vi "LJLogUD(old).vi"() -> ()   [LabVIEW 2020]
panel:
  in  "Change Working Directory":bool
  in  "Max File Size (Bytes)":i32=1048576 min=1 max=2000000000
  in  "Graph?":bool[](array[boolean])
  out "Waveform Graph":cluster{dbl, dbl, dbl[][]}(graph)
  in  "Graph History":i32=1000 min=0
  out "Address":string
  out "Device Type":string
  in  "Ranges":u16[](array[ring])=[0, 0, 0, 0, 0, 0, 0, 0] items=["LJ_rgBIP10V", "LJ_rgBIP5V", "LJ_rgUNI5V", "LJ_rgUNI2P5V", "LJ_rgUNI1P25V", "LJ_rgBIP1V", "LJ_rgUNIP625V", "LJ_rgBIPP1V", "LJ_rgBIPP01V"]
  in  "SettlingFactor":u8
  in  "Resolution":u8
  in  "exit":bool
  out "Scaled":dbl[](array[numeric]) format="%.6f"
  in  "Scaling Equation":string[](array[string])=["y=v0", "y=v1", "y=v2", "y=v3", "y=v4", "y=v5", "y=v6", "y=v7"]
  in  "# Channels":i32=4 min=1
  in  "-Ch":string[](array[string])=["31", "31", "31", "31", "31", "31", "31", "31"]
  out "Voltage":dbl[](array[numeric]) format="%.6f"
  in  "+Ch":string[](array[string])=["0", "1", "2", "3", "4", "5", "6", "7"]
  out "# of iterations":i32
  in  "Interval (ms)":u32=500
  out "Current Data File":path
  in  "Data File Prefix":string="data"
  in  "Write To File":bool
  out "Error Message":string
  # "0"
  # "1"
  # "2"
  # "3"
  # "4"
  # "5"
  # "6"
  # "7"
  # "8"
  # "9"
  # "10"
  # "11"
  # "12"
  # "13"
  # "14"
  # "15"
  # "-\"a\" - \"p\" correspond to the raw Voltage value\n  from the 1st through 16th row.\n-The scaled output value is \"y\".\n-If your equation has an error, the output\n  will be zero."
  # "# scans"
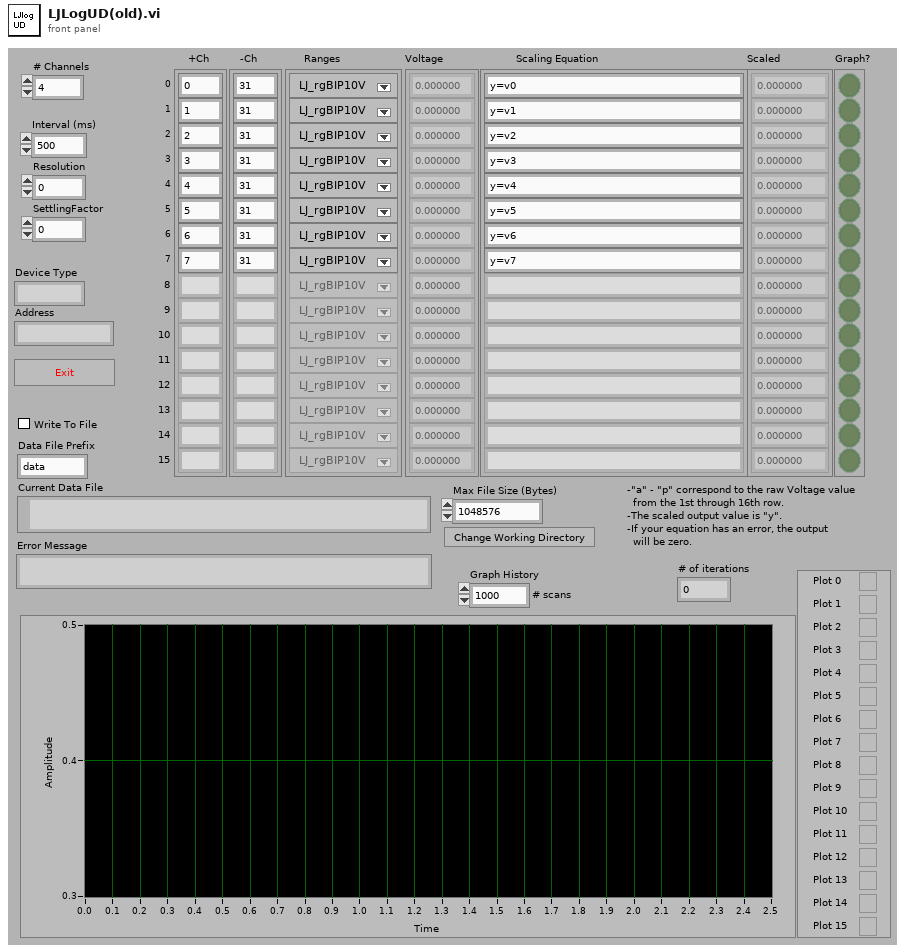
[diagram p1: front panel]
types:
  T1 = cluster{"+Ch":string[], "-Ch":string[], "Ranges":u16[], "Scaling Equation":string[], "Graph?":bool[]}
  T2 = cluster{"# Channels":i32, "+Ch":string[], "-Ch":string[], "Ranges":u16[], "Scaling Equation":string[]}
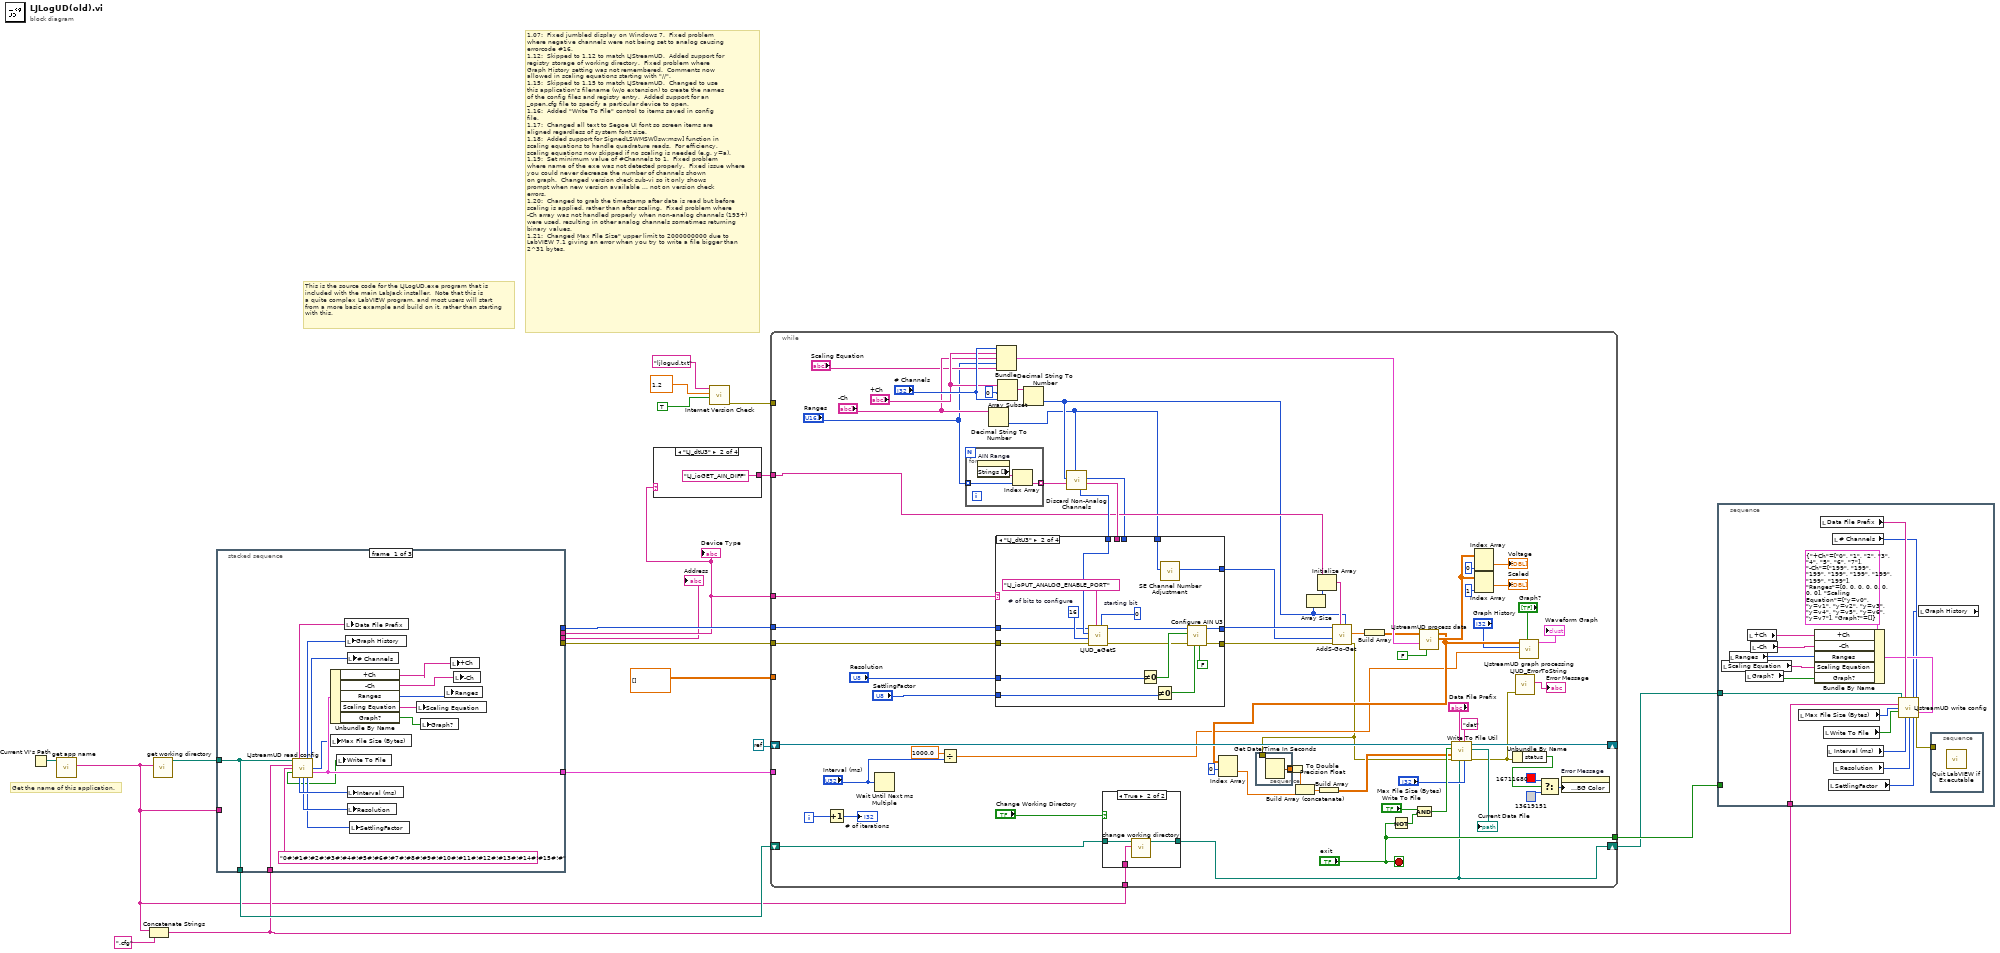
[diagram p0: block diagram]
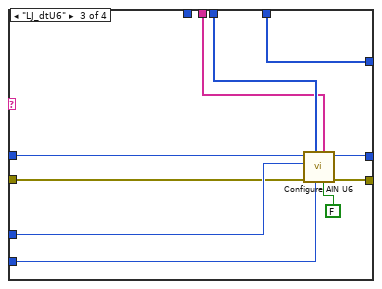
[diagram p4: hidden frame]
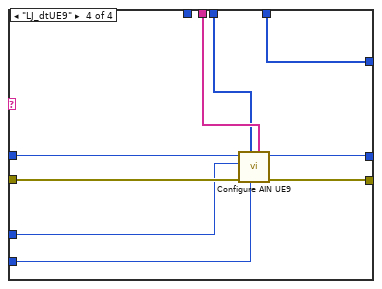
[diagram p5: hidden frame]
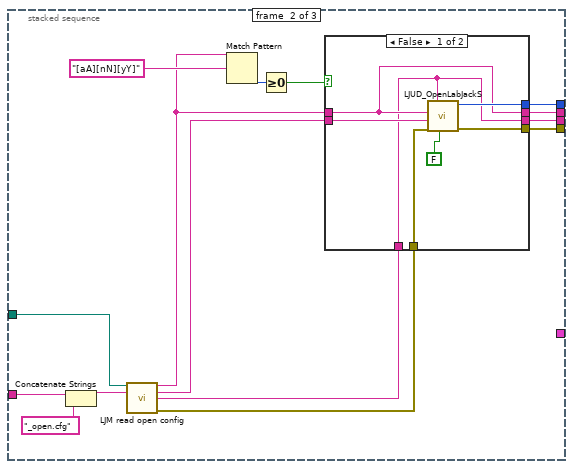
[diagram p6: hidden frame]
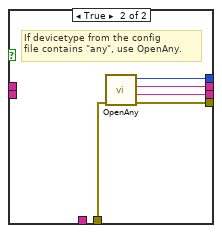
[diagram p7: hidden frame]
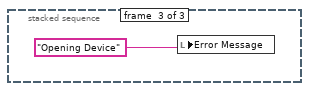
[diagram p8: hidden frame]
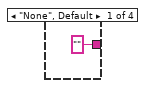
[diagram p9: hidden frame]
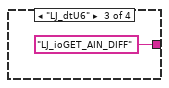
[diagram p10: hidden frame]
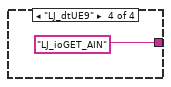
[diagram p11: hidden frame]
diagram:
  # "This is the source code for the LJLogUD.exe program that is\nincluded with the main LabJack installer.  Note that this is \na quite complex LabVIEW program, and most users will start\nfrom a more basic example and build on it, rather than starting\nwith this."
  # "Get the name of this application."
  # "1.07:  Fixed jumbled display on Windows 7.  Fixed problem\nwhere negative channels were not being set to analog causing\nerrorcode #16.\n1.12:  Skipped to 1.12 to match LJStreamUD.  Added support for\nregistry storage of working directory.  Fixed problem where\nGraph History setting was not remembered.  Comments now\nallowed in scaling equations starting with \"//\".\n1.15:  Skipped to 1.15 to match LJStreamUD.  Changed to use\nthis application's filename (w/o extension) to create the names\nof the config files and registry entry.  Added support for an\n_open.cfg file to specify a particular device to open.\n1.16:  Added \"Write To File\" control to items saved in config\nfile.\n1.17:  Changed all text to Segoe UI font so screen items are\naligned regardless of system font size.\n1.18:  Added support for SignedLSWMSW[lsw:msw] function in\nscaling equations to handle quadrature reads.  For efficiency,\nscaling equations now skipped if no scaling is needed (e.g. y=a).\n1.19:  Set minimum value of #Channels to 1.  Fixed problem\nwhere name of the exe was not detected properly.  Fixed issue where\nyou could never decrease the number of channels shown\non graph.  Changed version check sub-vi so it only shows\nprompt when new version available ... not on version check\nerrors.\n1.20:  Changed to grab the timestamp after data is read but before\nscaling is applied, rather than after scaling.  Fixed problem where\n-Ch array was not handled properly when non-analog channels (193+)\nwere used, resulting in other analog channels sometimes returning\nbinary values.\n1.21:  Changed Max File Size\" upper limit to 2000000000 due to\nLabVIEW 7.1 giving an error when you try to write a file bigger than\n2^31 bytes."
  n1 = Current VI's Path() -> (path=w1:path)
  n2 = call "get app name.vi"("Current VI's Path"=w1) -> ("App Name Without Extension"=w2:string)  [unwired: 4 in, 2 out]
  n3 = Concatenate Strings(w2, ".cfg" ("filename")) -> (w7:string)
  n4 = call "get working directory.vi"("Application Name"=w2) -> ("Working Directory"=w11:path)  [unwired: 9 in, 1 out]
  n5 = stacked-sequence {
    tunnel: [w37 _ _] -> w17
    tunnel: [w24 _ _] -> w10
    tunnel: w11 -> [w24 w38 _]
    tunnel: w7 -> [w23 _ _]
    tunnel: w2 -> [_ w51 _]
    tunnel: [_ w49 _] -> w6
    tunnel: [_ w48 _] -> w5
    tunnel: [_ w47 _] -> w4
    tunnel: [_ w46 _] -> w3
    frame #0 {
      n6 = call "LJstreamUD read config.vi"("Working Directory"=w24, "filename"=w23, "ChP Default"="0#!#1#!#2#!#3#!#4#!#5#!#6#!#7#!#8#!#9#!#10#!#11#!#12#!#13#!#14#!#15#!#") -> ("Data File Prefix"=w32:string, "Graph History"=w26:i32, "# Channels"=w28:i32, "Max File Size (Bytes)"=w25:i32, "Write To File"=w21:bool, "Channel Setup"=w37:T1, "Interval (ms)"=w31:u32, "Resolution"=w30:u8, "SettlingFactor"=w29:u8)  [unwired: 4 out]
      n7 = Unbundle By Name(w37) -> ("+Ch"=w33:string[], "-Ch"=w34:string[], "Ranges"=w35:u16[], "Scaling Equation"=w36:string[], "Graph?"=w27:bool[])
      n8 = local write "Max File Size (Bytes)"(w25) -> ()
      n9 = local write "Write To File"(w21) -> ()
      n10 = local write "Data File Prefix"(w32) -> ()
      n11 = local write "Graph History"(w26) -> ()
      n12 = local write "# Channels"(w28) -> ()
      n13 = local write "Interval (ms)"(w31) -> ()
      n14 = local write "Resolution"(w30) -> ()
      n15 = local write "SettlingFactor"(w29) -> ()
      n16 = local write "Scaling Equation"(w36) -> ()
      n17 = local write "Graph?"(w27) -> ()
      n18 = local write "Ranges"(w35) -> ()
      n19 = local write "+Ch"(w33) -> ()
      n20 = local write "-Ch"(w34) -> ()
    }
    frame #1 {
      n21 = Concatenate Strings(w51, "_open.cfg" ("filename")) -> (w50:string)
      n22 = call "LJM read open config.vi"("Working Directory"=w38, "filename"=w50) -> ("DeviceType"=w41:string, "ConnectionType"=w40:string, "Identifier"=w42:string, "error out"=w39:errorcluster)  [unwired: 10 in]
      n23 = Match Pattern(string=w41, regular expression="[aA][nN][yY]") -> (offset past match=w45:i32)  [unwired: 1 in, 3 out]
      n24 = Greater Or Equal To 0?(x=w45) -> (x >= 0?=w43:bool)
      n25 = case shown="False" w43 {
        tunnel: [w59 w64] -> w49
        tunnel: [w55 w63] -> w48
        tunnel: [w53 w62] -> w47
        tunnel: [w58 w61] -> w46
        tunnel: w42 -> [w53 _]
        tunnel: w41 -> [w55 _]
        tunnel: w40 -> [w54 _]
        tunnel: w39 -> [w56 w60]
        frame False {
          n26 = call "LJUD_OpenLabJackS.vi"("FirstFound"=FALSE, "Address"=w53, "error in"=w56, "ConnectionType"=w54, "DeviceType"=w55) -> ("error out"=w58:errorcluster, "Handle"=w59:i32)  [unwired: 4 in, 1 out]
        }
        frame True {
          # "If devicetype from the config\nfile contains \"any\", use OpenAny."
          n27 = call "OpenAny.vi"("error in"=w60) -> ("error out"=w61:errorcluster, "Address Found"=w62:string, "Device Type Found"=w63:string, "Handle"=w64:i32)  [unwired: 7 in]
        }
      }
    }
    frame #2 {
      n28 = local write "Error Message"("Opening Device" ("Error Message")) -> ()
    }
  }
  "Device Type" <- w5
  "Address" <- w4
  n29 = case shown="\"LJ_dtU3\"" w5 {
    tunnel: ["" ("IOType") "LJ_ioGET_AIN_DIFF" ("IOType") "LJ_ioGET_AIN_DIFF" ("IOType") "LJ_ioGET_AIN" ("IOType")] -> w19
    frame "None", Default {
    }
    frame "LJ_dtU3" {
    }
    frame "LJ_dtU6" {
    }
    frame "LJ_dtUE9" {
    }
  }
  n30 = call "Internet Version Check.vi"("Prompt If Newer Version Available"=TRUE, "Version In"=1.2, "Version File Name"="ljlogud.txt") -> ("error out"=w13:errorcluster)  [unwired: 6 in, 2 out]
  n31 = while {
    shift-left: w10 -> [w73]
    shift-right: [w72] -> w9
    tunnel: w2 -> [w74]
    tunnel: w13 -> [_]
    tunnel: dbl[][] [] ("Waveform Chart") -> [_]
    tunnel: w19 -> [w100]
    tunnel: w3 -> [w101]
    tunnel: w5 -> [w113]
    tunnel: w6 -> [w112]
    shift-left: refnum<k0> refnum -> [w122]
    shift-right: [w124] -> _
    tunnel: w17 -> [_]
    tunnel: ["exit"] -> w12
    i -> [w129]
    stop <- "exit" stop-if-true
    n32 = Increment(x=w129) -> (x+1=→"# of iterations":i32)
    n33 = Wait Until Next ms Multiple(millisecond multiple="Interval (ms)") -> ()  [unwired: 1 out]
    n34 = Divide(x=1000.0, y="Interval (ms)") -> (x/y=w85:dbl)
    n35 = for {
      tunnel: "Ranges" -> [w184] mode=indexing
      tunnel: [w183] -> w130 mode=indexing
      n36 = property on="AIN Range" class="Ring (strict)"() -> ("Strings []"=w185:string[])  [unwired: 2 in, 2 out]
      n37 = Index Array(array=w185, index=w184) -> (element=w183:string)
    }
    n38 = Decimal String To Number(string="-Ch") -> (number=w70:i32[])  [unwired: 2 in, 1 out]
    n39 = Bundle("# Channels"="# Channels", "+Ch"="+Ch", "-Ch"="-Ch", "Ranges"="Ranges", "Scaling Equation"="Scaling Equation") -> (w117:T2)  [unwired: 1 in]
    n40 = Array Subset(array="+Ch", index=0 ("Array Index"), length="# Channels") -> (w131:string[])
    n41 = Decimal String To Number(string=w131) -> (number=w81:i32[])  [unwired: 2 in, 1 out]
    n42 = call "Discard Non-Analog Channels.vi"("Channels In (-)"=w70, "Ranges In"=w130, "Channels In"=w81) -> ("Ranges Out"=w110:string[], "Channels Out"=w82:i32[], "FIO/EIO Analog Enable"=w111:i32)  [unwired: 5 in, 1 out]
    n43 = case shown="\"LJ_dtU3\"" w113 {
      tunnel: w111 -> [_ w152 _ _]
      tunnel: w101 -> [w146 w151 w165 w181]
      tunnel: w112 -> [w145 w150 w166 w182]
      tunnel: [w146 w158 w172 w177] -> w106
      tunnel: [w145 w159 w173 w178] -> w104
      tunnel: w110 -> [_ _ w170 w180]
      tunnel: w82 -> [_ _ w171 w179]
      tunnel: "Resolution" -> [_ w163 w169 w176]
      tunnel: "SettlingFactor" -> [_ w161 w168 w175]
      tunnel: [w144 w157 w164 w174] -> w103
      tunnel: w70 -> [w144 w147 w164 w174]
      frame "None", Default {
      }
      frame "LJ_dtU3" {
        w154 = 0  # starting bit
        w155 = 16  # # of bits to configure
        n44 = call "LJUD_eGetS.vi"("Channel"=w154, "IOType"="LJ_ioPUT_ANALOG_ENABLE_PORT" ("Channel"), "error in"=w151, "x1"=w155, "Value Write"=w152, "Handle In"=w150) -> ("error out"=w149:errorcluster, "Handle Out"=w148:i32)  [unwired: 3 in, 1 out]
        n45 = Not Equal To 0?(x=w163) -> (x != 0?=w162:bool)
        n46 = Not Equal To 0?(x=w161) -> (x != 0?=w160:bool)
        n47 = call "SE Channel Number Adjustment.vi"("Channels In"=w147) -> ("Channels Out"=w157:i32[])  [unwired: 10 in]
        n48 = call "Configure AIN U3.vi"("Binary"=FALSE ("Enable DAC1"), "longSettling"=w160, "error in"=w149, "quickSample"=w162, "Handle In"=w148) -> ("error out"=w158:errorcluster, "Handle Out"=w159:i32)  [unwired: 5 in]
      }
      frame "LJ_dtU6" {
        n49 = call "Configure AIN U6.vi"("Binary"=FALSE ("Enable Counter0"), "Ranges"=w170, "SettlingFactor"=w168, "Positive Channels"=w171, "error in"=w165, "Resolution"=w169, "Handle In"=w166) -> ("error out"=w172:errorcluster, "Handle Out"=w173:i32)  [unwired: 3 in]
      }
      frame "LJ_dtUE9" {
        n50 = call "Configure AIN UE9.vi"("Ranges"=w180, "SettlingFactor"=w175, "Channels"=w179, "error in"=w181, "Resolution"=w176, "Handle In"=w182) -> ("error out"=w177:errorcluster, "Handle Out"=w178:i32)  [unwired: 4 in]
      }
    }
    n51 = case shown="True" "Change Working Directory" {
      tunnel: w74 -> [_ w141]
      tunnel: w73 -> [w138 w140]
      tunnel: [w138 w139] -> w72
      frame False {
      }
      frame True {
        n52 = call "change working directory.vi"("Application Name"=w141, "Working Directory In"=w140) -> ("Working Directory Out"=w139:path)  [unwired: 9 in]
      }
    }
    n53 = Array Size(array=w81) -> (size(s)=w115:i32)
    n54 = Initialize Array(w100, w115) -> (w114:string[])
    n55 = call "AddS-Go-Get.vi"("Channels"=w81, "IOTypes"=w114, "error in"=w106, "x1"=w103, "Handle In"=w104) -> ("error out"=w71:errorcluster, "Values Read"=w105:dbl[])  [unwired: 4 in, 1 out]
    n56 = stacked-sequence {
      tunnel: [w143] -> w99
      tunnel: w71 -> [_]
      frame #0 {
        n57 = Get Date/Time In Seconds() -> (seconds since 1Jan1904=w142:timestamp)
        n58 = To Double Precision Float(number=w142) -> (double precision float=w143:dbl)
      }
    }
    n59 = Build Array(w105) -> (w97:dbl[][])
    n60 = Not(x="exit") -> (.not. x?=w133:bool)
    n61 = And(x="Write To File", y=w133) -> (x .and. y?=w123:bool)
    n62 = call "LJstreamUD process data.vi"("Disable Scaling"=FALSE, "Channel Config"=w117, "Voltages"=w97) -> ("Volts,Scaled Averages"=w116:dbl[][], "Scaled Data"=w90:dbl[][])  [unwired: 7 in]
    n63 = Index Array(array=w90, index (row)=0 ("Index (row)")) -> (element=w95:dbl[])  [unwired: 1 in]
    n64 = Build Array (concatenate)(w99, w95) -> (w98:dbl[])
    n65 = Build Array(w98) -> (w94:dbl[][])
    n66 = call "Write To File Util.vi"("Maximum File Size (Bytes)"="Max File Size (Bytes)", "Data File Extension"="dat", "Working Directory"=w72, "Data File Prefix"="Data File Prefix", "error in"=w71, "Data"=w94, "Write To File"=w123, "File Refnum In"=w122) -> ("error out"=w80:errorcluster, "Current Data File"=→"Current Data File":path, "File Refnum Out"=w124:refnum<file>)  [unwired: 1 in]
    n67 = Index Array(array=w116, index (col)=0 ("Disabled Index (col)")) -> (element=→"Voltage":dbl[])  [unwired: 1 in]
    n68 = Index Array(array=w116, index (col)=1 ("Disabled Index (col)")) -> (element=→"Scaled":dbl[])  [unwired: 1 in]
    n69 = Unbundle By Name(w80) -> ("status"=w79:bool)
    n70 = call "LJUD_ErrorToString.vi"("error in"=w80) -> ("String"=→"Error Message":string)  [unwired: 10 in]
    n71 = call "LJstreamUD graph processing.vi"("Graph?"="Graph?", "Scan Rate"=w85, "Graph History (# scans)"="Graph History", "Scaled Data"=w90) -> ("Graph Data"=→"Waveform Graph":cluster{dbl, dbl, dbl[][]})  [unwired: 7 in]
    n72 = Select(t=u32 16711680, s=w79, f=u32 13619151) -> (s? t:f=w78:u32)
    n73 = property on="Error Message" class="Str"("Text.Text Colors:BG Color"=w78) -> ()  [unwired: 2 in, 2 out]
  }
  n74 = stacked-sequence {
    tunnel: w9 -> [w190]
    tunnel: w12 -> [_]
    tunnel: w7 -> [w187]
    frame #0 {
      n75 = local read "Scaling Equation"() -> (w194:string[])
      n76 = local read "Ranges"() -> (w195:u16[])
      n77 = local read "Graph?"() -> (w193:bool[])
      n78 = local read "+Ch"() -> (w197:string[])
      n79 = local read "-Ch"() -> (w196:string[])
      n80 = local read "Max File Size (Bytes)"() -> (w189:i32)
      n81 = Bundle By Name(cluster=T1 {"+Ch"=["0", "1", "2", "3", "4", "5", "6", "7"], "-Ch"=["199", "199", "199", "199", "199", "199", "199", "199"], "Ranges"=[0, 0, 0, 0, 0, 0, 0, 0], "Scaling Equation"=["y=v0", "y=v1", "y=v2", "y=v3", "y=v4", "y=v5", "y=v6", "y=v7"], "Graph?"=[]} ("Channel Setup"), "+Ch"=w197, "-Ch"=w196, "Ranges"=w195, "Scaling Equation"=w194, "Graph?"=w193) -> (w192:T1)
      n82 = local read "Data File Prefix"() -> (w202:string)
      n83 = local read "Write To File"() -> (w186:bool)
      n84 = local read "Interval (ms)"() -> (w201:u32)
      n85 = local read "SettlingFactor"() -> (w199:u8)
      n86 = local read "# Channels"() -> (w191:i32)
      n87 = local read "Resolution"() -> (w200:u8)
      n88 = local read "Graph History"() -> (w188:i32)
      n89 = call "LJstreamUD write config.vi"("Working Directory"=w190, "Data File Prefix"=w202, "Graph History"=w188, "# Channels"=w191, "filename"=w187, "Max File Size (Bytes)"=w189, "Write To File"=w186, "Channel Setup"=w192, "Interval (ms)"=w201, "Resolution"=w200, "SettlingFactor"=w199) -> ("error out"=w203:errorcluster)  [unwired: 4 in]
      n90 = stacked-sequence {
        tunnel: w203 -> [_]
        frame #0 {
          n91 = call "Quit LabVIEW if Executable.vi"() -> ()  [unwired: 1 in]
        }
      }
    }
  }
